vi "Read Controller Type.vi"(8 "error in (no error)":errorcluster, 11 "Generic Controller in":refnum<class "Generic Plugin.lvclass">) -> (0 "error out":errorcluster, 2 "Controller Type":T1, 3 "Generic Controller out":refnum<class "Generic Plugin.lvclass">)   [LabVIEW 2020, in "Generic Plugin.lvclass"]
uses:
  Generic Plugin.lvclass
  Controller Type.ctl
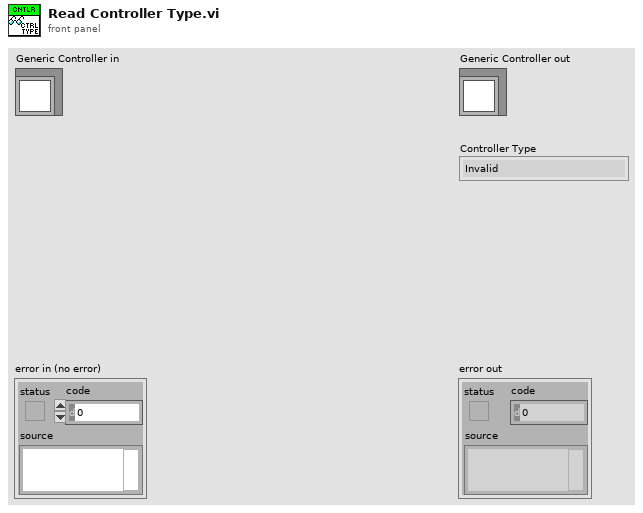
[diagram p1: front panel]
types:
  T1 = typedef "Generic Plugin.lvclass/Controller Type.ctl" = enum16{"Invalid", "Temperature Controller", "Pump Controller", "Generic Optimizer", "LC Parser"}
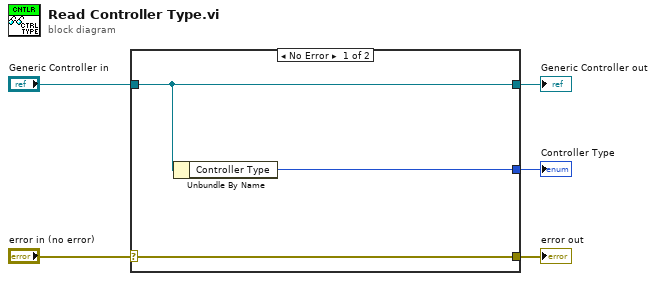
[diagram p0: block diagram]
diagram:
  n1 = case shown="No Error" "error in (no error)" {
    selector: "error in (no error)" -> [w8 w9]
    tunnel: [w8 w9] -> w4
    tunnel: [w7 w10] -> w2
    tunnel: "Generic Controller in" -> [w7 w10]
    tunnel: [w6 _] -> w1
    frame No Error {
      n2 = Unbundle By Name(w7) -> ("Controller Type"=w6:T1)
    }
    frame Error {
    }
  }
  "error out" <- w4
  "Generic Controller out" <- w2
  "Controller Type" <- w1
